vi "_word.bookmark.text.vi"(7 "Application":refnum<k7>, 8 "error IO":errorcluster, 11 "Bookmark":refnum<k7>) -> (0 "error out":errorcluster, 2 "Text":string, 3 "Bookmark(dup)":refnum<k7>)   [LabVIEW 2018, in "WordReportGeneration.lvlib"]
uses:
  WordReportGeneration.lvlib
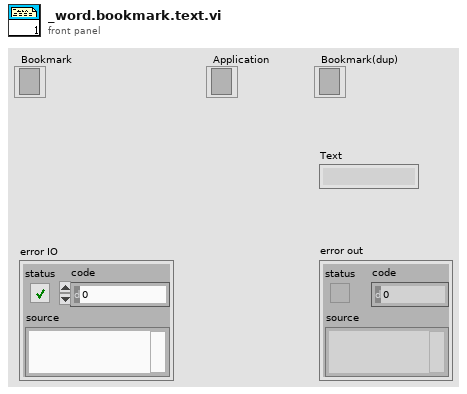
[diagram p1: front panel]
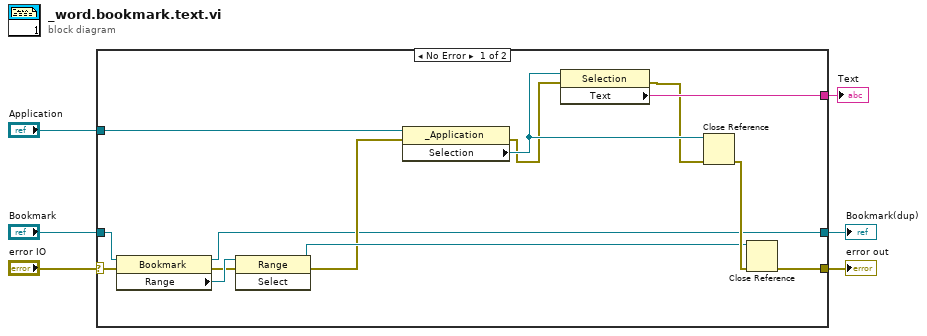
[diagram p0: block diagram]
diagram:
  n1 = case shown="No Error" "error IO" {
    selector: "error IO" -> [w19 w22]
    tunnel: [w20 w22] -> w6
    tunnel: [w13 w21] -> w4
    tunnel: "Application" -> [w12 _]
    tunnel: "Bookmark" -> [w11 w21]
    tunnel: [w9 _] -> w1
    frame No Error {
      n2 = property class="Bookmark"(reference=w11, error in=w19) -> (reference out=w13:refnum<k7>, error out=w15:errorcluster, "Range"=w18:refnum<k7>)
      n3 = invoke class="Range" method="Select"(reference=w18, error in=w15) -> (reference out=w16:refnum<k7>, error out=w14:errorcluster)  [unwired: 1 in, 1 out]
      n4 = property class="_Application"(reference=w12, error in=w14) -> (error out=w8:errorcluster, "Selection"=w10:refnum<k7>)  [unwired: 1 out]
      n5 = property class="Selection"(reference=w10, error in=w8) -> (error out=w7:errorcluster, "Text"=w9:string)  [unwired: 1 out]
      n6 = Close Reference(reference=w10, error in (no error)=w7) -> (error out=w17:errorcluster)
      n7 = Close Reference(reference=w16, error in (no error)=w17) -> (error out=w20:errorcluster)
    }
    frame Error {
    }
  }
  "error out" <- w6
  "Bookmark(dup)" <- w4
  "Text" <- w1
